vi "test bin file.vi"() -> ()   [LabVIEW 2013, in "Binary logger tests.lvlib"]
uses:
  Binary logger tests.lvlib
  <vilib>/NI/Tag Bus/dictionary/data dictionary.lvclass/data dictionary.ctl
  execution/data cache.ctl
  <vilib>/NI/Tag Bus/table/data table.ctl
  <vilib>/NI/Configuration Framework/serializable configuration/NISE_CEF_serializable configuration.lvclass
  execution/Binary datalogger runtime.lvclass
  <vilib>/NI/Tag Bus/dictionary/data dictionary.lvclass
  <vilib>/NI/Tag Bus/table/data table.lvlib
panel:
  out "empty?":bool
  out "x = y? 3":bool
  out "x = y? 2":bool
  out "x = y?":bool
  out "del error":errorcluster
  out "error out":errorcluster
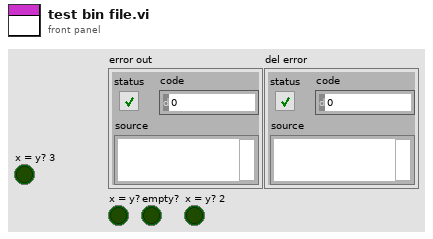
[diagram p1: front panel]
types:
  T1 = enum16{"open", "replace", "create", "open or create", "replace or create", "replace or create with confirmation"}
  T2 = typedef "tag bus.lvlib/data dictionary.lvclass/full data dictionary.ctl" = cluster{"Double":string[], "Single":string[], "I64":string[], "I32":string[], "I16":string[], "I8":string[], "U64":string[], "U32":string[], "U16":string[], "U8":string[], "Boolean":string[], "String":string[], "Array of Double":string[], "Array of Single":string[], "Array of I64":string[], "Array of I32":string[], "Array of I16":string[], "Array of I8":string[], "Array of U64":string[], "Array of U32":string[], "Array of U16":string[], "Array of U8":string[], "Array of Boolean":string[], "Array of String":string[]}
  T3 = typedef "tag bus.lvlib/data table.lvlib/data table.ctl" = cluster{"Double":dbl[], "Single":sgl[], "I64":i64[], "I32":i32[], "I16":i16[], "I8":i8[], "U64":u64[], "U32":u32[], "U16":u16[], "U8":u8[], "Boolean":bool[], "String":string[], "Array of Double":cluster{"DBL Array":dbl[]}[], "Array of Single":cluster{"SGL Array":sgl[]}[], "Array of I64":cluster{"I64 Array":i64[]}[], "Array of I32":cluster{"I32 Array":i32[]}[], "Array of I16":cluster{"I16 Array":i16[]}[], "Array of I8":cluster{"I8 Array":i8[]}[], "Array of U64":cluster{"U64 Array":u64[]}[], "Array of U32":cluster{"U32 Array":u32[]}[], "Array of U16":cluster{"U16 Array":u16[]}[], "Array of U8":cluster{"U8 Array":u8[]}[], "Array of Boolean":cluster{"Boolean Array":bool[]}[], "Array of String":cluster{"String Array":string[]}[]}
  T4 = typedef "Binary datalogger runtime.lvclass/data cache.ctl" = cluster{"timestamps":timestamp[], "dataset":T3[]}
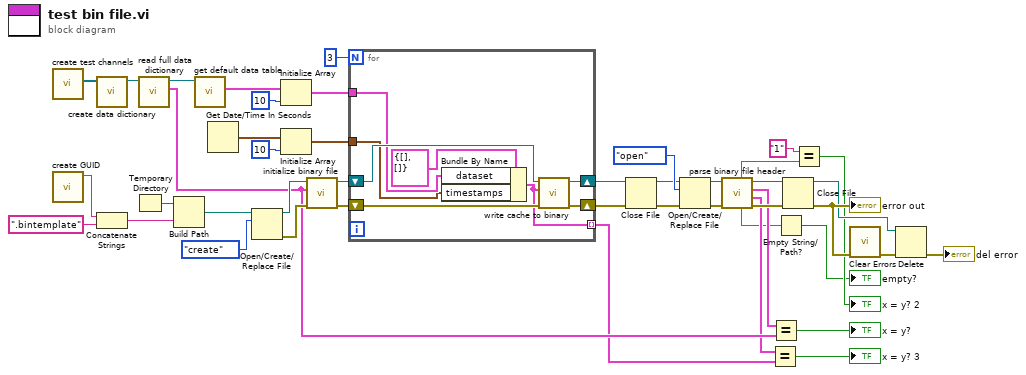
[diagram p0: block diagram]
diagram:
  n1 = call "create test channels.vi"() -> ("chans"=w16:refnum<class "TBM channel.lvclass">[])  [unwired: 8 in, 3 out]
  n2 = call <vilib>:"create GUID.vi"() -> ("uuid"=w43:string)  [unwired: 10 in, 1 out]
  n3 = call <vilib>:"create data dictionary.vi"("system tags"=w16) -> ("data dictionary"=w15:refnum<class "data dictionary.lvclass">)  [unwired: 9 in, 1 out]
  n4 = Concatenate Strings(w43, ".bintemplate" ("string")) -> (w41:string)
  n5 = Temporary Directory() -> (w44:path)
  n6 = call <vilib>:"read full data dictionary.vi"("data dictionary in"=w15) -> ("dictionary"=w14:T2, "data dictionary out"=w13:refnum<class "data dictionary.lvclass">)  [unwired: 8 in, 1 out]
  n7 = Build Path(base path=w44, name or relative path=w41) -> (appended path=w40:path)
  n8 = call <vilib>:"get default data table.vi"("data dictionary in"=w13) -> ("default data table"=w12:T3)  [unwired: 9 in, 1 out]
  n9 = Get Date/Time In Seconds() -> (seconds since 1Jan1904=w9:timestamp)
  n10 = Open/Create/Replace File(file path (use dialog)=w40, operation (0:open)=T1."create") -> (refnum out=w38:refnum<file>, error out=w37:errorcluster)  [unwired: 4 in, 1 out]
  n11 = Initialize Array(w12, 10 ("dimension size")) -> (w8:T3[])
  n12 = Initialize Array(w9, 10 ("dimension size")) -> (w7:timestamp[])
  n13 = call "initialize binary file.vi"("error in"=w37, "dictionary"=w14, "Byte Stream File in"=w38) -> ("error out"=w17:errorcluster, "Byte Stream File out"=w20:refnum<file>)  [unwired: 7 in]
  n14 = for {
    N: 3 -> [_]
    shift-right: [w51] -> w19
    shift-left: w20 -> [w52]
    shift-right: [w50] -> w18
    shift-left: w17 -> [w49]
    tunnel: w8 -> [w47]
    tunnel: w7 -> [w46]
    tunnel: [w45] -> w4 mode=indexing
    n15 = Bundle By Name(cluster=T4 {"timestamps"=[], "dataset"=[]} ("cache in"), "dataset"=w47, "timestamps"=w46) -> (w45:T4)
    n16 = call "write cache to binary.vi"("error in"=w49, "cache in"=w45, "bin file in"=w52) -> ("error out"=w50:errorcluster, "bin file out"=w51:refnum<file>)  [unwired: 6 in, 1 out]
  }
  n17 = Close File(refnum=w19, error in=w18) -> (path=w35:path, error out=w34:errorcluster)
  n18 = Open/Create/Replace File(file path (use dialog)=w35, error in=w34, operation (0:open)=T1."open") -> (refnum out=w29:refnum<file>, error out=w26:errorcluster)  [unwired: 3 in, 1 out]
  n19 = call "parse binary file header.vi"("error in"=w26, "Byte Stream File in"=w29) -> ("error out"=w27:errorcluster, "data"=w3:T4[], "dictionary"=w25:T2, "Byte Stream File out"=w28:refnum<file>, "remaining string"=w2:string, "version"=w23:string)  [unwired: 4 in]
  n20 = Equal?(x=w3, y=w4) -> (x = y?=→"x = y? 3":bool)
  n21 = Equal?(x=w25, y=w14) -> (x = y?=→"x = y?":bool)
  n22 = Empty String/Path?(string/path=w2) -> (empty?=→"empty?":bool)
  n23 = Close File(refnum=w28, error in=w27) -> (path=w32:path, error out=w33:errorcluster)
  "error out" <- w33
  n24 = Equal?(x="1", y=w23) -> (x = y?=→"x = y? 2":bool)
  n25 = call <vilib>:"Clear Errors.vi"("error in (no error)"=w33) -> ("error out"=w31:errorcluster)  [unwired: 6 in]
  n26 = Delete(path (use dialog)=w32, error in=w31) -> (error out=→"del error":errorcluster)  [unwired: 3 in, 2 out]
